vi "sub_map-data_all.vi"() -> (3 "map-data_all":T1(array[cluster]))   [LabVIEW 2019]
uses:
  Ctrl/gps-databuf.ctl
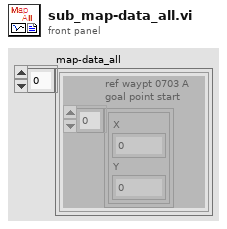
[diagram p1: front panel]
types:
  T1 = cluster{"ref waypt 0703 A \ngoal point start":cluster{"X":dbl, "Y":dbl}[]}[]
  T2 = typedef "gps-databuf.ctl" = enum16{"read", "write"}
  T3 = cluster{"rawdata":string, "GPS Data":cluster{"Latitude":cluster{"Valid?":bool, "Latitude (Deg)":dbl}, "Longitude":cluster{"Valid?":bool, "Longitude (Deg)":dbl}, "Height":cluster{"Valid?":bool, "Height (m)":dbl}, "Undulation":cluster{"Valid?":bool, "Undulation(m)":dbl}, "North Vel":cluster{"Valid?":bool, "North Vel (m/s)":dbl}, "East Vel":cluster{"Valid?":bool, "East Vel (m/s)":dbl}, "Up Vel":cluster{"Valid?":bool, "Up Vel (m/s)":dbl}, "Roll":cluster{"Valid?":bool, "Roll (degrees)":dbl}, "Pitch":cluster{"Valid?":bool, "Pitch (degrees)":dbl}, "Azimuth":cluster{"Valid?":bool, "Azimuth (degrees)":dbl}, "Lat deviation":cluster{"Valid?":bool, "Lat deviation (m)":dbl}, "Long deviation":cluster{"Valid?":bool, "Long deviation (m)":dbl}, "Height deviation":cluster{"Valid?":bool, "Height deviation (m)":dbl}, "North vel deviation":cluster{"Valid?":bool, "North vel deviation (m/s)":dbl}, "East vel deviation":cluster{"Valid?":bool, "East vel deviation (m/s)":dbl}, "Up vel deviation":cluster{"Valid?":bool, "Up vel deviation (m/s)":dbl}, "Roll deviation":cluster{"Valid?":bool, "Roll deviation (degrees)":dbl}, "Pitch deviation":cluster{"Valid?":bool, "Pitch deviation (degrees)":dbl}, "Azimuth deviation":cluster{"Valid?":bool, "Azimuth deviation (degrees)":dbl}, "Ext sol status":cluster{"Valid?":bool, "Ext sol status":dbl}}, "Heading":dbl, "utm-1":cluster{"XN":dbl, "YE":dbl}}
  T4 = cluster{"ref waypt 0703 A \ngoal point start":cluster{"X":dbl, "Y":dbl}[]}
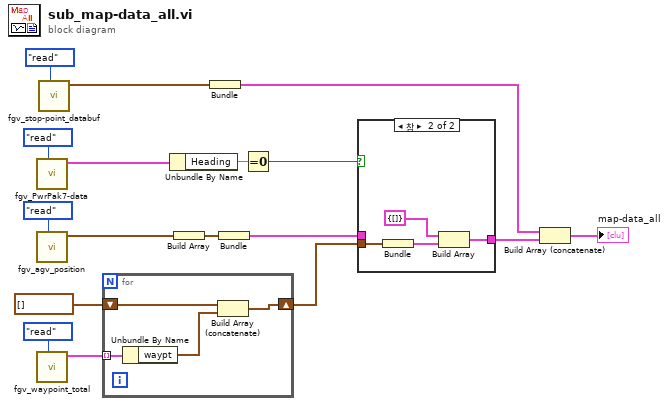
[diagram p0: block diagram]
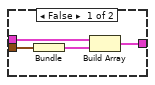
[diagram p2: hidden frame]
diagram:
  n1 = call "fgv_PwrPak7-data.vi"("cmd"=gps-databuf."read") -> ("data cluster out"=w8:T3)  [unwired: 9 in, 1 out]
  n2 = call "fgv_agv_position.vi"("cmd"=enum16{"write", "read"}."read") -> ("agv curr utm out"=w5:cluster{dbl, dbl})  [unwired: 8 in, 2 out]
  n3 = call "fgv_waypoint_total.vi"("cmd"=enum16{"write", "read"}."read") -> ("waypoint total out"=w2:cluster{"waypt":cluster{"X":dbl, "Y":dbl}[]}[])  [unwired: 10 in]
  n4 = call "fgv_stop-point_databuf.vi"("cmd"=enum16{"clear", "write", "read"}."read") -> ("all stop pts out"=w14:cluster{dbl, dbl}[])  [unwired: 10 in]
  n5 = for {
    shift-right: [w19] -> w3
    shift-left: cluster{"X":dbl, "Y":dbl}[] [] ("ref waypt 0703 A \ngoal point start") -> [w21]
    tunnel: w2 -> [w20] mode=indexing
    n6 = Unbundle By Name(w20) -> ("waypt"=w18:cluster{"X":dbl, "Y":dbl}[])
    n7 = Build Array (concatenate)(w21, w18) -> (w19:cluster{"X":dbl, "Y":dbl}[])
  }
  n8 = Unbundle By Name(w8) -> ("Heading"=w9:dbl)
  n9 = Build Array(w5) -> (w6:cluster{dbl, dbl}[])
  n10 = Bundle("all stop pts out"=w14) -> (w17:cluster{"all stop pts out":cluster{dbl, dbl}[]})  [unwired: 1 in]
  n11 = Bundle(w6) -> (w7:cluster{cluster{dbl, dbl}[]})  [unwired: 1 in]
  n12 = Equal To 0?(x=w9) -> (x = 0?=w11:bool)
  n13 = case shown="참" w11 {
    tunnel: w3 -> [w23 w28]
    tunnel: [w25 w29] -> w13
    tunnel: w7 -> [w24 _]
    frame False {
      n14 = Bundle("ref waypt 0703 A \ngoal point start"=w23) -> (w22:T4)  [unwired: 1 in]
      n15 = Build Array(w24, w22) -> (w25:T1)
    }
    frame True {
      n16 = Bundle("ref waypt 0703 A \ngoal point start"=w28) -> (w27:T4)  [unwired: 1 in]
      n17 = Build Array(T4 {"ref waypt 0703 A \ngoal point start"=[]}, w27) -> (w29:T1)
    }
  }
  n18 = Build Array (concatenate)(w17, w13) -> (→"map-data_all":T1)
